vi "GetDataFlowScript.vi"(8 "error in (no error)":errorcluster, 11 "type":T1) -> (0 "error out":errorcluster, 2 "found":bool, 3 "Dataflow script":string[](array[string]))   [LabVIEW 2017, in "DataFlow.lvlib"]
uses:
  <vilib>/addons/InsightCM/Devices/Shared/Common/DataFlow/DataFlow.lvlib
  <vilib>/addons/InsightCM/Devices/Shared/Common/DataFlow/controls/Type.ctl
  <vilib>/addons/PointValueMap/subVIs/Point_Read_variant.vi
  <vilib>/addons/InsightCM/Utilities/GlobalConfiguration/GlobalConfiguration.lvlib
  <vilib>/addons/PointValueMap/PointValueMap.lvlib
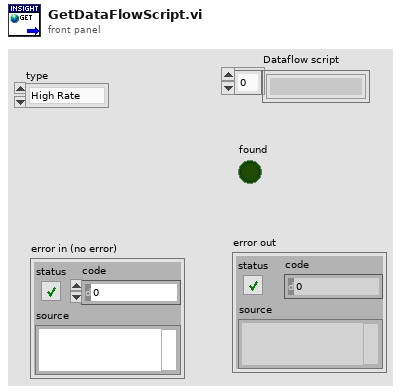
[diagram p1: front panel]
types:
  T1 = typedef "DataFlow.lvlib/Type.ctl" = enum16{"High Rate", "Low Rate", "Burst Mode"}
  T2 = typedef "PointValueMap.lvlib/PointMap.ctl" = refnum<data-value>
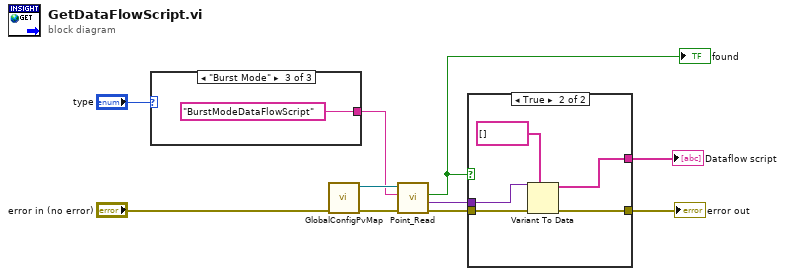
[diagram p0: block diagram]
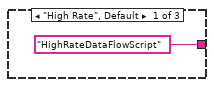
[diagram p2: hidden frame]
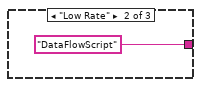
[diagram p3: hidden frame]
diagram:
  n1 = case shown="\"Burst Mode\"" "type" {
    tunnel: ["HighRateDataFlowScript" ("Name") "DataFlowScript" ("Name") "BurstModeDataFlowScript" ("Name")] -> w1
    frame "High Rate", Default {
    }
    frame "Low Rate" {
    }
    frame "Burst Mode" {
    }
  }
  n2 = call <vilib>:"GlobalConfigPvMap.vi"("error in (no error)"="error in (no error)") -> ("error out"=w10:errorcluster, "global configuration map"=w9:T2)  [unwired: 9 in]
  n3 = call-poly <vilib>:"Point_Read.vi"("Error In"=w10, "Tag"=w1, "Map"=w9) -> ("Error Out"=w7:errorcluster, "Value"=w5:variant, "Found?"=w3:bool)  [unwired: 3 in, 3 out]
  "found" <- w3
  n4 = case shown="True" w3 {
    tunnel: w7 -> [w14 w18]
    tunnel: [w14 w17] -> w6
    tunnel: w5 -> [_ w16]
    tunnel: [_ w15] -> w4
    frame False {
    }
    frame True {
      n5 = Variant To Data(error in=w18, type=string[] [] ("DataFlow"), Variant=w16) -> (data=w15:string[], error out=w17:errorcluster)
    }
  }
  "error out" <- w6
  "Dataflow script" <- w4
